vi "DecodeBase64ToLVImage.vi"(8 "error in (no error)":errorcluster, 11 "Base64String":string) -> (0 "error out":errorcluster, 3 "LVImage":T1)   [LabVIEW 2020]
doc: "Decode a Base64 Image string to an LV Image"
uses:
  <vilib>/picture/picture.llb/imagedata.ctl
  <vilib>/Utility/error.llb/Error Cluster From Error Code.vi
  <vilib>/ErrorRing/Error Ring.xnode
  <vilib>/wsapi/NI_WebServices.lvlib
  <vilib>/JDP Science/JDP Science Common Utilities/Base64/Base64 Support.lvlib
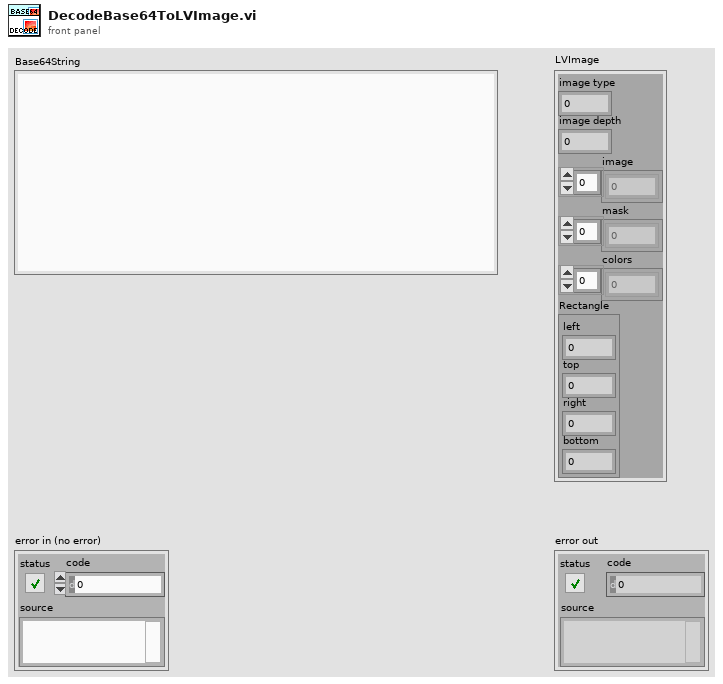
[diagram p1: front panel]
types:
  T1 = typedef "imagedata.ctl" = cluster{"image type":i32, "image depth":i32, "image":u8[], "mask":u8[], "colors":u32[], "Rectangle":cluster{"left":i16, "top":i16, "right":i16, "bottom":i16}}
  T2 = enum16{"open", "replace", "create", "open or create", "replace or create", "replace or create with confirmation"}
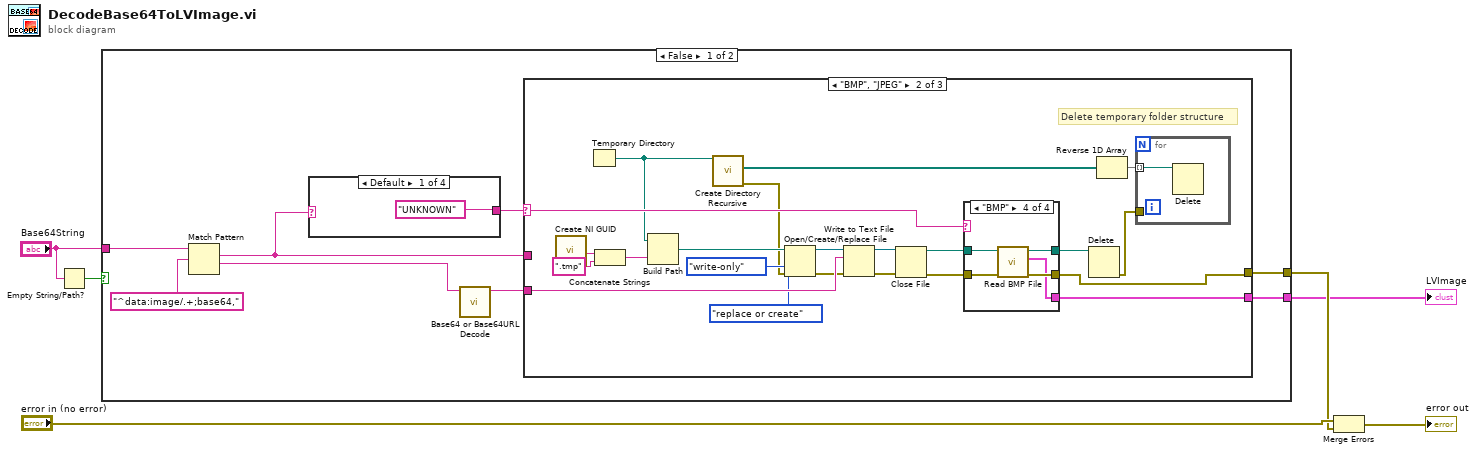
[diagram p0: block diagram]
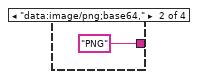
[diagram p2: hidden frame]
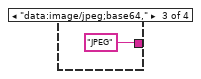
[diagram p3: hidden frame]
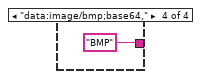
[diagram p4: hidden frame]
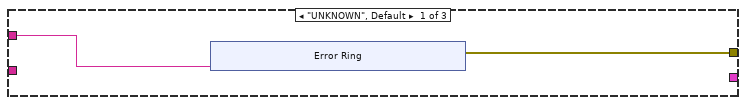
[diagram p5: hidden frame]
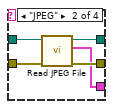
[diagram p7: hidden frame]
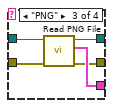
[diagram p8: hidden frame]
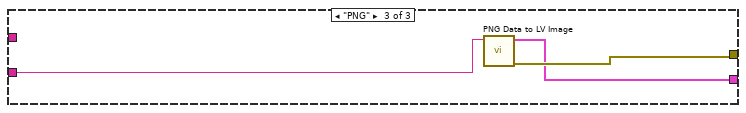
[diagram p9: hidden frame]
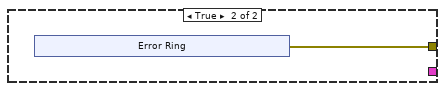
[diagram p10: hidden frame]
diagram:
  n1 = Empty String/Path?(string/path="Base64String") -> (empty?=w1:bool)
  n2 = case shown="False" w1 {
    tunnel: [w14 w71] -> w4
    tunnel: "Base64String" -> [w12 _]
    tunnel: [w7 _] -> w3
    frame False {
      n3 = Match Pattern(string=w12, regular expression="^data:image/.+;base64,") -> (match substring=w11:string, after substring=w10:string)  [unwired: 1 in, 2 out]
      n4 = case shown="Default" w11 {
        tunnel: ["UNKNOWN" "PNG" "JPEG" "BMP"] -> w8
        frame Default {
        }
        frame "data:image/png;base64," {
        }
        frame "data:image/jpeg;base64," {
        }
        frame "data:image/bmp;base64," {
        }
      }
      n5 = call <vilib>:"Base64 or Base64URL Decode.vi"("Base64 or Base64URL"=w10) -> ("Decoded"=w9:string)  [unwired: 10 in]
      n6 = case shown="\"BMP\", \"JPEG\"" w8 {
        selector: w8 -> [_ w39 _]
        tunnel: [w20 w33 w70] -> w14
        tunnel: w11 -> [w19 _ _]
        tunnel: w9 -> [_ w41 w68]
        tunnel: [_ w40 w69] -> w7
        frame "UNKNOWN", Default {
          n7 = xnode "Error Ring"("parameter 0"=w19) -> ("error out"=w20:errorcluster)
        }
        frame "BMP", "JPEG" {
          # "Delete temporary folder structure"
          n8 = call <vilib>:"Create NI GUID.vi"() -> ("NI GUID"=w43:string)
          n9 = Temporary Directory() -> (w31:path)
          n10 = Concatenate Strings(w43, ".tmp" ("string")) -> (w44:string)
          n11 = Build Path(base path=w31, name or relative path=w44) -> (appended path=w38:path)
          n12 = call <vilib>:"Create Directory Recursive.vi"("directory"=w31) -> ("error out"=w32:errorcluster, "directories created"=w28:path[])  [unwired: 4 in, 1 out]
          n13 = Open/Create/Replace File(file path (use dialog)=w38, error in=w32, operation (0:open)=T2."replace or create", access (0:read/write)=enum16{"read/write", "read-only", "write-only"}."write-only") -> (refnum out=w37:refnum<file>, error out=w35:errorcluster)  [unwired: 2 in, 1 out]
          n14 = Write to Text File(file (use dialog)=w37, text=w41, error in=w35) -> (refnum out=w46:refnum<file>, error out=w45:errorcluster)  [unwired: 1 in, 1 out]
          n15 = Close File(refnum=w46, error in=w45) -> (path=w48:path, error out=w49:errorcluster)
          n16 = case shown="\"BMP\"" w39 {
            tunnel: [w52 w57 w61 w66] -> w47
            tunnel: w48 -> [w52 w56 w62 w67]
            tunnel: w49 -> [w51 w55 w58 w63]
            tunnel: [w51 w54 w59 w65] -> w33
            tunnel: [_ w53 w60 w64] -> w40
            frame Default {
            }
            frame "JPEG" {
              n17 = call <vilib>:"Read JPEG File.vi"("error in (no error)"=w55, "path to JPEG file"=w56) -> ("error out"=w54:errorcluster, "image data"=w53:T1, "path"=w57:path)  [unwired: 7 in]
            }
            frame "PNG" {
              n18 = call <vilib>:"Read PNG File.vi"("error in (no error)"=w58, "path to PNG file"=w62) -> ("error out"=w59:errorcluster, "image data"=w60:T1, "path"=w61:path)  [unwired: 7 in]
            }
            frame "BMP" {
              n19 = call <vilib>:"Read BMP File.vi"("error in (no error)"=w63, "path to BMP file"=w67) -> ("error out"=w65:errorcluster, "image data"=w64:T1, "path"=w66:path)  [unwired: 7 in]
            }
          }
          n20 = Delete(path (use dialog)=w47) -> (error out=w29:errorcluster)  [unwired: 4 in, 2 out]
          n21 = Reverse 1D Array(array=w28) -> (reversed array=w30:path[])
          n22 = for {
            tunnel: w30 -> [w50] mode=indexing
            tunnel: w29 -> [_]
            n23 = Delete(path (use dialog)=w50) -> ()  [unwired: 4 in, 3 out]
          }
        }
        frame "PNG" {
          n24 = call <vilib>:"PNG Data to LV Image.vi"("png data"=w68) -> ("error out"=w70:errorcluster, "image data"=w69:T1)  [unwired: 9 in]
        }
      }
    }
    frame True {
      n25 = xnode "Error Ring"() -> ("error out"=w71:errorcluster)
    }
  }
  "LVImage" <- w3
  n26 = Merge Errors("error in (no error)", w4) -> (→"error out":errorcluster)
